vi "Initialize.vi"(8 "Error In":errorcluster, 11 "Size":i32) -> (0 "Error Out":errorcluster, 2 "return type":i32, 3 "Map id":i32)   [LabVIEW 2018]
uses:
  <vilib>/Utility/error.llb/Error Cluster From Error Code.vi
  <vilib>/ErrorRing/Error Ring.xnode
  SharedMemoryTest.dll
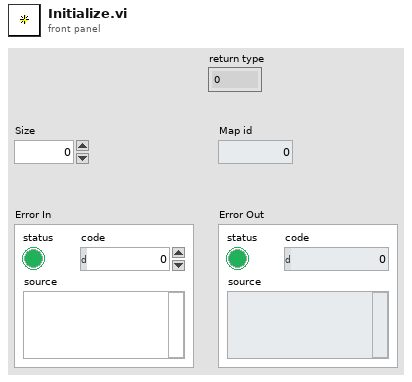
[diagram p1: front panel]
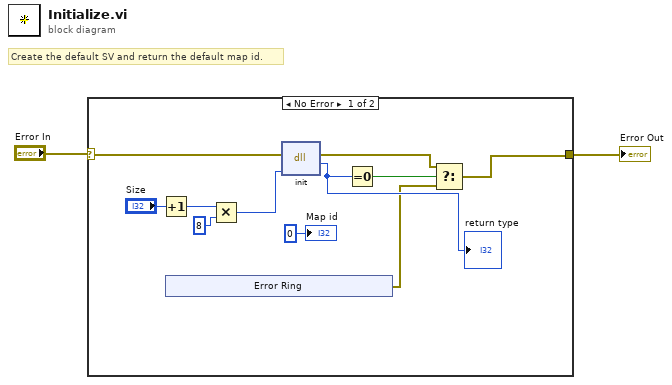
[diagram p0: block diagram]
diagram:
  # "Create the default SV and return the default map id."
  n1 = case shown="No Error" "Error In" {
    selector: "Error In" -> [w13 w18]
    tunnel: [w4 w18] -> w1
    frame No Error {
      n2 = Increment(x="Size") -> (x+1=w9:i32)
      n3 = xnode "Error Ring"() -> ("error out"=w3:errorcluster)
      n4 = Multiply(x=w9, y=8) -> (x*y=w8:i32)
      n5 = dll-call lib="C:/Users/jaros/Desktop/UIF_StateVector/SV operations/SharedMemoryTest.dll" fn="init"(error in=w13, "size"=w8) -> (error out=w5:errorcluster, "return type"=w7:i32)  [unwired: 3 in, 1 out]
      "return type" <- w7
      n6 = Equal To 0?(x=w7) -> (x = 0?=w6:bool)
      n7 = Select(t=w5, s=w6, f=w3) -> (s? t:f=w4:errorcluster)
      "Map id" <- 0 ("Map id")
    }
    frame Error {
    }
  }
  "Error Out" <- w1
